vi "JoinGroupCommands.vi"(8 "error in (no error)":errorcluster, 9 "Seperator":string[](array[string]), 11 "Msg in":T1) -> (0 "error out":errorcluster, 1 "Seperator out":string=".Channel", 3 "Msg out":T1)   [LabVIEW 2011]
uses:
  DriverMsg.ctl
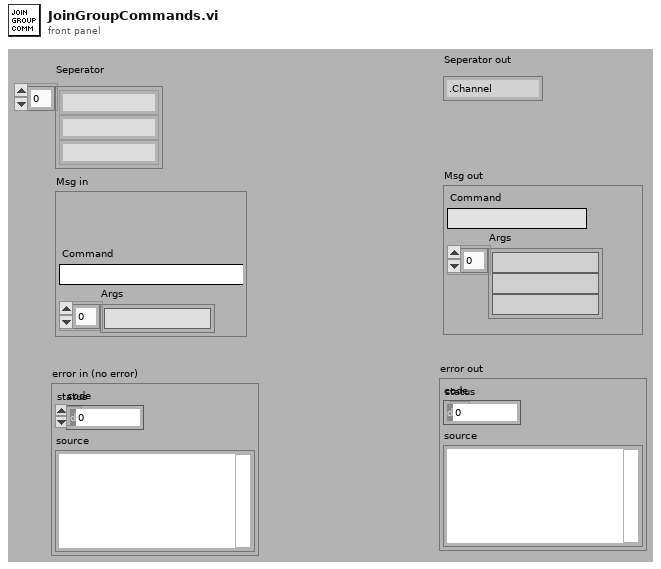
[diagram p1: front panel]
types:
  T1 = typedef "DriverMsg.ctl" = cluster{"Command":string, "Args":string[]}
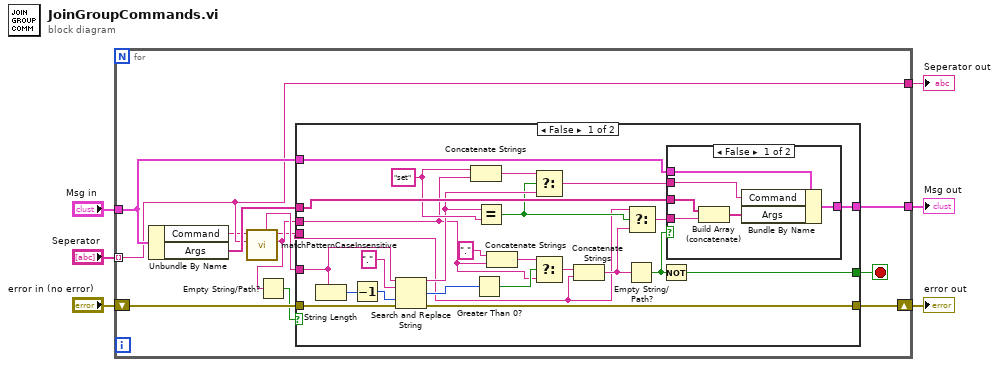
[diagram p0: block diagram]
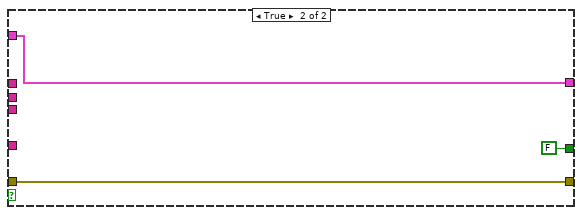
[diagram p3: hidden frame]
diagram:
  n1 = for {
    tunnel: [w18] -> w6
    tunnel: [w12] -> w5
    shift-right: [w16] -> w4
    shift-left: "error in (no error)" -> [w15]
    tunnel: "Msg in" -> [w14]
    tunnel: "Seperator" -> [w12] mode=indexing
    stop <- w13 stop-if-true
    n2 = Unbundle By Name(w14) -> ("Command"=w11:string, "Args"=w17:string[])
    n3 = call "matchPatternCaseInsensitive.vi"("String"=w12, "Command 4"=w11) -> ("match"=w9:string, "after"=w7:string, "before"=w10:string)  [unwired: 7 in]
    n4 = Empty String/Path?(string/path=w9) -> (empty?=w8:bool)
    n5 = case shown="False" w8 {
      tunnel: [w43 w53] -> w18
      tunnel: w17 -> [w42 _]
      tunnel: [w27 w51] -> w16
      tunnel: w15 -> [w26 w51]
      tunnel: w14 -> [w25 w53]
      tunnel: [w23 FALSE] -> w13
      tunnel: w7 -> [w22 _]
      tunnel: w10 -> [w21 _]
      tunnel: w9 -> [w19 _]
      frame False {
        w34 = "set" ("y")
        n6 = String Length(string=w21) -> (length=w20:i32)
        n7 = Decrement(x=w20) -> (x-1=w38:i32)
        n8 = Search and Replace String(input string=w21, search string=".", offset=w38, error in=w26) -> (result string=w33:string, number of replacements=w37:i32, error out=w27:errorcluster)  [unwired: 4 in, 1 out]
        n9 = Concatenate Strings(w34, w19) -> (w31:string)
        n10 = Greater Than 0?(x=w37) -> (x > 0?=w36:bool)
        n11 = Equal?(x=w33, y=w34) -> (x = y?=w30:bool)
        n12 = Concatenate Strings("." ("x"), w19) -> (w41:string)
        n13 = Select(t=w31, s=w30, f=w33) -> (s? t:f=w32:string)
        n14 = Select(t=w41, s=w36, f=w19) -> (s? t:f=w40:string)
        n15 = Concatenate Strings(w40, w22) -> (w29:string)
        n16 = Empty String/Path?(string/path=w29) -> (empty?=w24:bool)
        n17 = Select(t=w22, s=w30, f=w29) -> (s? t:f=w28:string)
        n18 = Not(x=w24) -> (.not. x?=w23:bool)
        n19 = case shown="False" w24 {
          tunnel: w25 -> [w49 w50]
          tunnel: [w48 w50] -> w43
          tunnel: w32 -> [w47 _]
          tunnel: w42 -> [w46 _]
          tunnel: w28 -> [w44 _]
          frame False {
            n20 = Build Array (concatenate)(w46, w44) -> (w45:string[])
            n21 = Bundle By Name(cluster=w49, "Command"=w47, "Args"=w45) -> (w48:T1)
          }
          frame True {
          }
        }
      }
      frame True {
      }
    }
  }
  "Msg out" <- w6
  "Seperator out" <- w5
  "error out" <- w4
